vi "Method_Const.vi"(4 "Value":dbl, 5 "Abs_Waveform.lvclass":refnum<class "Abs_Waveform.lvclass">) -> (1 "Result":refnum<class "Abs_Waveform.lvclass">)   [LabVIEW 2021, in "Subtract_WFM_Numeric.lvclass"]
uses:
  Subtract_WFM_Numeric.lvclass
  Abs_Types/Waveform/Abs_Waveform.lvclass
  C:/TSA/LV_Abstract/Source/Functions/Support/Function/Two Terminal/WFM_Numeric/AbsFunc_Two Term_WFM_Numeric.lvclass
  C:/Program Files (x86)/National Instruments/LabVIEW 2021/vi.lib/TSA/Abstract Data Classes/Abs_Types/Waveform/Abs_Waveform.lvclass
  Support/Function/Two Terminal/WFM_Numeric/AbsFunc_Two Term_WFM_Numeric.lvclass/AbsFunc_Two Term_WFM_Numeric.ctl
  Support/Function/Two Terminal/WFM_Numeric/Properties/Write Abs_Waveform.lvclass.vi
  Support/Function/Two Terminal/WFM_Numeric/Properties/Write Numeric.lvclass.vi
  Constants/Support/DBL/Const_DBL.lvclass
  C:/Program Files (x86)/National Instruments/LabVIEW 2021/vi.lib/TSA/Abstract Data Classes/Abs_Types/Numeric/Abs_Numeric.lvclass
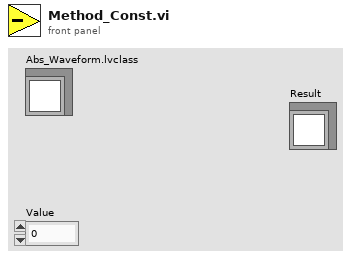
[diagram p1: front panel]
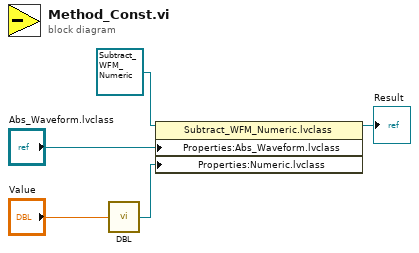
[diagram p0: block diagram]
diagram:
  n1 = call "DBL.vi"("Value"="Value") -> ("Constant"=w2:refnum<class "Const_DBL.lvclass">)  [unwired: 4 in]
  n2 = property class="Subtract_WFM_Numeric.lvclass"(reference=refnum<class "Subtract_WFM_Numeric.lvclass"> refnum ("Functions.lvlib:Numeric.lvlib:Add_DBL.lvclass"), "Properties:Abs_Waveform.lvclass"="Abs_Waveform.lvclass", "Properties:Numeric.lvclass"=w2) -> (reference out=→"Result":refnum<class "Subtract_WFM_Numeric.lvclass">)  [unwired: 1 in, 1 out]
